vi "GUI.vi"() -> ()   [LabVIEW 2021]
uses:
  <vilib>/numeric/Random Number (Range) U64.vi
  <vilib>/numeric/sub_Random U32.vi
  <vilib>/Instr/_visa.llb/VISA Configure Serial Port (Instr).vi
panel:
  out "start sim":bool
  out "Time has Elapsed":bool
  out "Time":dbl
  out "Logging":bool caption="Time has Elapsed"
  in  "PWM":i16(slide)=1410 min=1300 max=1410 scale=1155.0..1384.0
  out "Mode":string
  in  "Mode":bool
  out "O":dbl
  out "T":dbl
  out "D":dbl
  out "I":dbl
  out "P":dbl
  out "F":dbl
  out "S":dbl
  in  "Stop Button":bool
  out "TS":dbl(slide) scale=0.0..100.0
  out "KD":dbl(slide) scale=0.0..100.0
  out "KI":dbl(slide) scale=0.0..50.0
  out "KP":dbl(slide) scale=0.0..10.0
  in  "COM Port":refnum<visa-resource-name>
  in  "Save Result":path
  out "Output PID":dbl(graph)
  out "Tacho Generator":dbl(knob) scale=0.0..1023.0
  out "SetPoint":dbl(knob) scale=0.0..1023.0
  out "Respon PID":dynamicdata(graph)
  # "ALIM SATRIA FI'I WIJAYA KUSUMA (21/483503/SV/20304)"
  # "KENDALI KECEPATAN MOTOR DC"
  # "ILHAM DWI CAHYO (21/483417/SV/20218)"
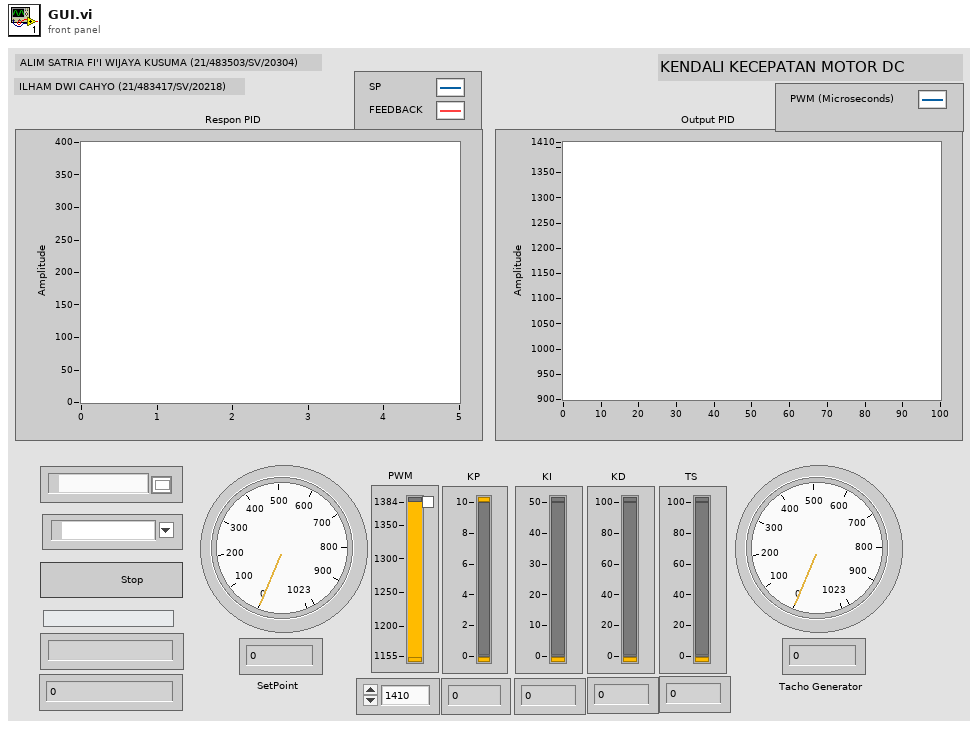
[diagram p1: front panel]
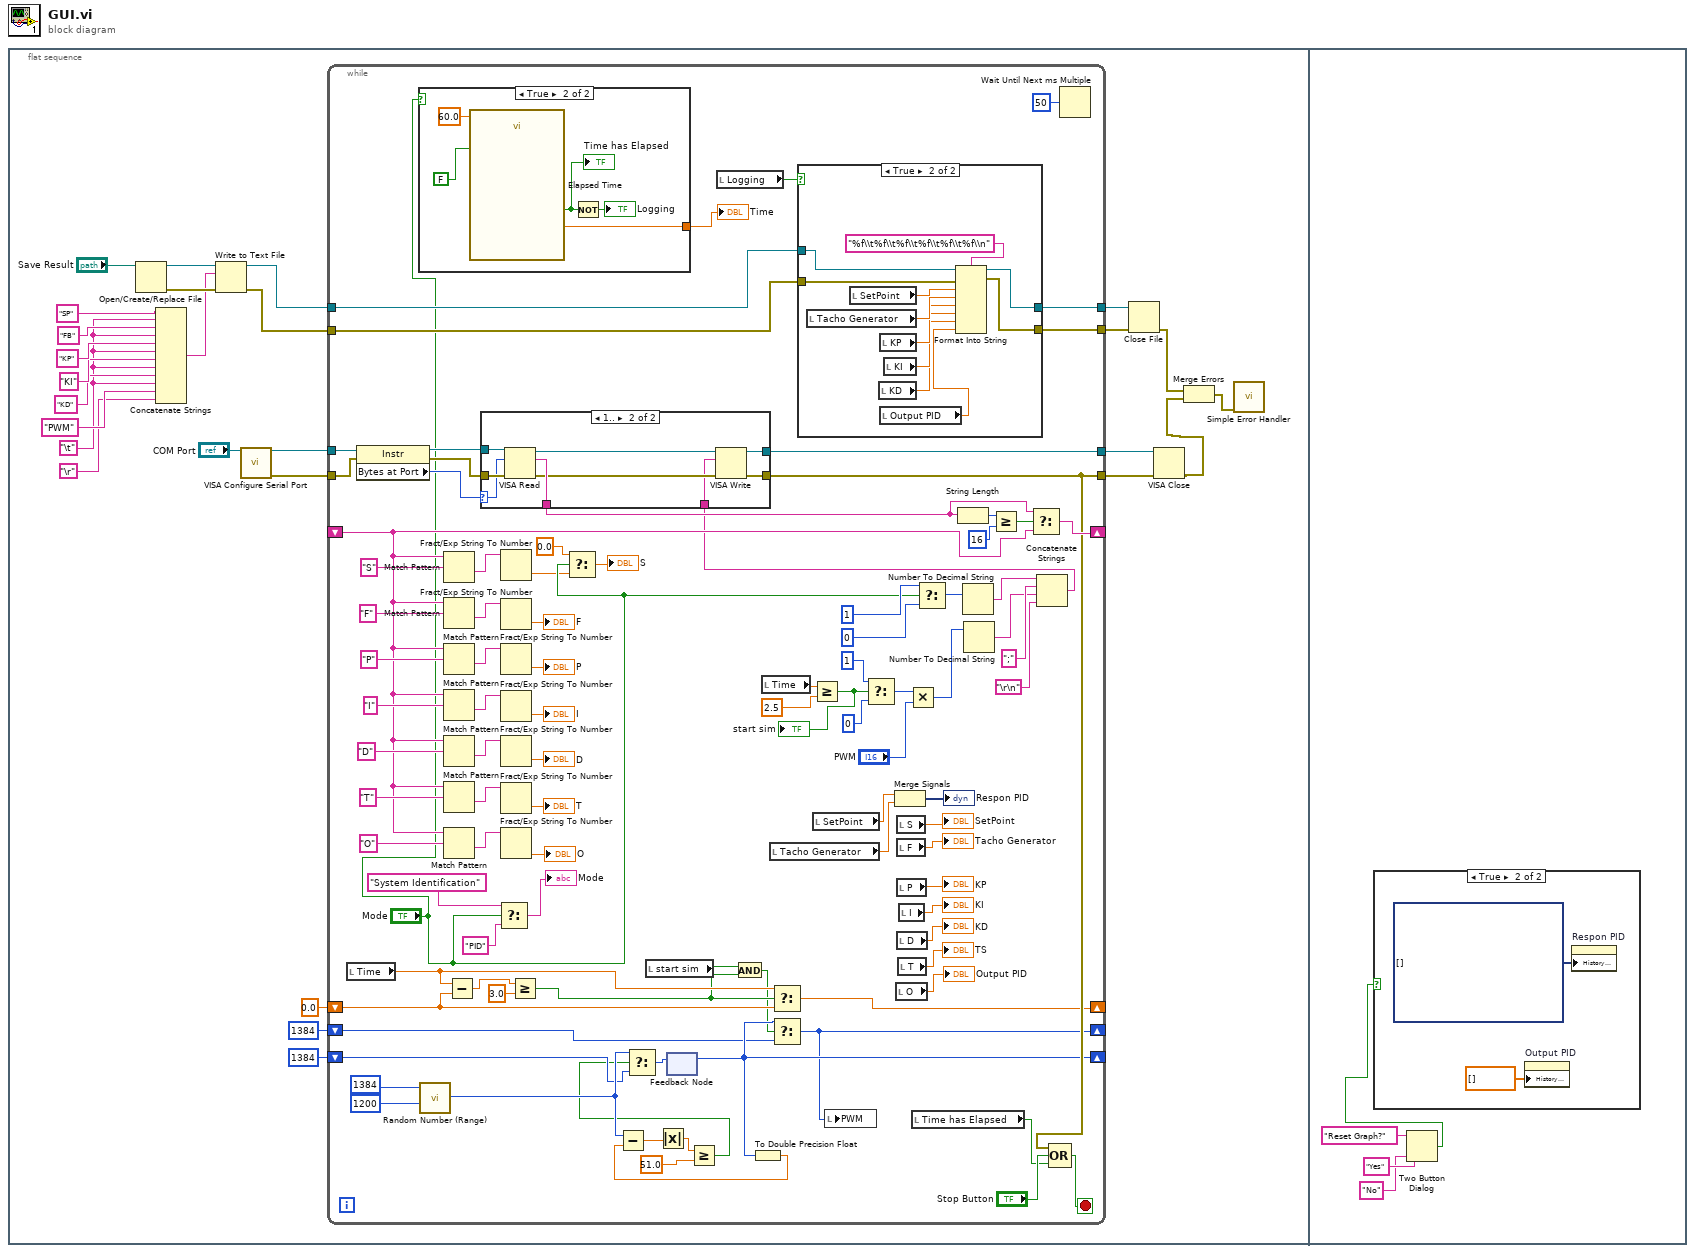
[diagram p0: block diagram]
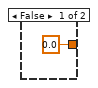
[diagram p2: hidden frame]
diagram:
  n1 = flat-sequence {
    frame #0 {
      w10 = "\t"
      n2 = Open/Create/Replace File(file path (use dialog)="Save Result") -> (refnum out=w22:refnum<file>, error out=w23:errorcluster)  [unwired: 5 in, 1 out]
      n3 = Concatenate Strings("SP", w10, "FB" ("string"), w10, "KP" ("string"), w10, "KI" ("string"), w10, "KD" ("string"), w10, "PWM", "\r") -> (w17:string)
      n4 = Write to Text File(file (use dialog)=w22, text=w17, error in=w23) -> (refnum out=w21:refnum<file>, error out=w20:errorcluster)  [unwired: 1 in, 1 out]
      n5 = call-poly "VISA Configure Serial Port"("VISA resource name"="COM Port") -> ("VISA resource name out"=w27:refnum<visa-resource-name>, "error out"=w26:errorcluster)  [unwired: 13 in]
      n6 = while {
        tunnel: w27 -> [w83]
        tunnel: w26 -> [w79]
        tunnel: [w80] -> w8
        tunnel: [w74] -> w7
        tunnel: w21 -> [w93]
        tunnel: w20 -> [w92]
        tunnel: [w91] -> w19
        tunnel: [w90] -> w18
        shift-right: [w86] -> _
        shift-left: _ -> [w85]
        shift-right: [w33] -> _
        shift-left: u64 1384 ("number") -> [w35]
        shift-right: [w40] -> _
        shift-left: 0.0 ("Time") -> [w36]
        shift-right: [w31] -> _
        shift-left: u64 1384 ("number") -> [w32]
        stop <- w124 stop-if-true
        n7 = local read "Time"() -> (w37:dbl)
        n8 = property class="Instr"(reference=w83, error in=w79) -> (reference out=w82:refnum<visa-resource-name>, error out=w81:errorcluster, "Bytes at Port"=w123:u32)
        n9 = case shown="True" "Mode" {
          tunnel: [0.0 ("Elapsed Time (s)") w127] -> w63
          frame False {
          }
          frame True {
            n10 = call "Elapsed Time"("Time Target (s)"=60.0, "Auto Reset"=FALSE) -> ("Elapsed Time (s)"=w127:dbl, "Time has Elapsed"=w130:bool)  [unwired: 10 in, 6 out]
            "Time has Elapsed" <- w130
            n11 = Not(x=w130) -> (.not. x?=→"Logging":bool)
          }
        }
        "Time" <- w63
        n12 = call-poly <vilib>:"Random Number (Range).vi"("lower bound (0)"=u64 1200, "upper bound (100)"=u64 1384) -> ("number"=w47:u64)  [unwired: 9 in]
        n13 = Match Pattern(string=w85, regular expression="S") -> (after substring=w115:string)  [unwired: 1 in, 3 out]
        n14 = Match Pattern(string=w85, regular expression="F") -> (after substring=w114:string)  [unwired: 1 in, 3 out]
        n15 = Match Pattern(string=w85, regular expression="P") -> (after substring=w113:string)  [unwired: 1 in, 3 out]
        n16 = Match Pattern(string=w85, regular expression="I") -> (after substring=w112:string)  [unwired: 1 in, 3 out]
        n17 = Match Pattern(string=w85, regular expression="D") -> (after substring=w111:string)  [unwired: 1 in, 3 out]
        n18 = Match Pattern(string=w85, regular expression="T") -> (after substring=w110:string)  [unwired: 1 in, 3 out]
        n19 = Match Pattern(string=w85, regular expression="O") -> (after substring=w109:string)  [unwired: 1 in, 3 out]
        n20 = Subtract(x=w37, y=w36) -> (x-y=w38:dbl)
        n21 = Select(t="System Identification", s="Mode", f="PID") -> (s? t:f=→"Mode":string)
        n22 = Fract/Exp String To Number(string=w115) -> (number=w52:dbl)  [unwired: 3 in, 1 out]
        n23 = Fract/Exp String To Number(string=w114) -> (number=→"F":dbl)  [unwired: 3 in, 1 out]
        n24 = Fract/Exp String To Number(string=w113) -> (number=→"P":dbl)  [unwired: 3 in, 1 out]
        n25 = Fract/Exp String To Number(string=w112) -> (number=→"I":dbl)  [unwired: 3 in, 1 out]
        n26 = Fract/Exp String To Number(string=w111) -> (number=→"D":dbl)  [unwired: 3 in, 1 out]
        n27 = Fract/Exp String To Number(string=w110) -> (number=→"T":dbl)  [unwired: 3 in, 1 out]
        n28 = Fract/Exp String To Number(string=w109) -> (number=→"O":dbl)  [unwired: 3 in, 1 out]
        n29 = Greater Or Equal?(x=w38, y=3.0) -> (x >= y?=w29:bool)
        n30 = Select(t=0.0, s="Mode", f=w52) -> (s? t:f=→"S":dbl)
        n31 = local read "start sim"() -> (w30:bool)
        n32 = feedback #1() -> (w33:u64)  [unwired: 1 in]
        n33 = local read "Logging"() -> (w64:bool)
        n34 = And(x=w30, y=w29) -> (x .and. y?=w28:bool)
        n35 = To Double Precision Float(number=w33) -> (double precision float=w43:dbl)
        n36 = Subtract(x=w47, y=w43) -> (x-y=w45:dbl)
        n37 = Absolute Value(x=w45) -> (abs(x)=w46:dbl)
        n38 = Greater Or Equal?(x=w46, y=51.0) -> (x >= y?=w34:bool)
        n39 = Select(t=w47, s=w34, f=w35) -> (s? t:f=w44:u64)
        n40 = feedback-in #1(w44) -> ()
        n41 = local read "Time"() -> (w61:dbl)
        n42 = local read "Tacho Generator"() -> (w101:dbl)
        n43 = Select(t=w37, s=w29, f=w36) -> (s? t:f=w40:dbl)
        n44 = Select(t=w33, s=w28, f=w32) -> (s? t:f=w31:u64)
        n45 = case shown="True" w64 {
          tunnel: w93 -> [w132 w143]
          tunnel: w92 -> [w131 w142]
          tunnel: [w132 w141] -> w91
          tunnel: [w131 w140] -> w90
          frame False {
          }
          frame True {
            n46 = local read "Tacho Generator"() -> (w138:dbl)
            n47 = local read "SetPoint"() -> (w139:dbl)
            n48 = local read "KD"() -> (w134:dbl)
            n49 = local read "KP"() -> (w136:dbl)
            n50 = local read "Output PID"() -> (w133:dbl)
            n51 = local read "KI"() -> (w135:dbl)
            n52 = Format Into String(format string="%f\\t%f\\t%f\\t%f\\t%f\\t%f\\n", initial string=w143, error in=w142, w139, w138, w136, w135, w134, w133) -> (resulting string=w141:refnum<file>, error out=w140:errorcluster)
          }
        }
        n53 = Greater Or Equal?(x=w61, y=2.5) -> (x >= y?=w59:bool)
        "start sim" <- w59
        n54 = local read "SetPoint"() -> (w102:dbl)
        n55 = local write "PWM"(w31) -> ()
        n56 = Select(t=i16 1, s=w59, f=i16 0) -> (s? t:f=w56:i16)
        n57 = Merge Signals(w102, w101) -> (→"Respon PID":dynamicdata)
        n58 = local read "O"() -> (→"Output PID":dbl)
        n59 = local read "S"() -> (→"SetPoint":dbl)
        n60 = local read "F"() -> (→"Tacho Generator":dbl)
        n61 = local read "P"() -> (→"KP":dbl)
        n62 = local read "D"() -> (→"KD":dbl)
        n63 = local read "T"() -> (→"TS":dbl)
        n64 = local read "I"() -> (→"KI":dbl)
        n65 = Multiply(x=w56, y="PWM") -> (x*y=w54:i16)
        n66 = local read "Time has Elapsed"() -> (w62:bool)
        n67 = Select(t=1, s="Mode", f=0) -> (s? t:f=w66:i32)
        n68 = Number To Decimal String(number=w66) -> (decimal integer string=w70:string)  [unwired: 1 in]
        n69 = Number To Decimal String(number=w54) -> (decimal integer string=w69:string)  [unwired: 1 in]
        n70 = Concatenate Strings(w70, ";", w69, "\r\n") -> (w73:string)
        n71 = case shown="1.." w123 {
          selector: w123 -> [_ w151]
          tunnel: w82 -> [w145 w154]
          tunnel: [w145 w148] -> w80
          tunnel: w81 -> [w144 w153]
          tunnel: [w144 w147] -> w74
          tunnel: [_ w152] -> w84
          tunnel: w73 -> [_ w146]
          frame 0, Default {
          }
          frame 1.. {
            n72 = VISA Read(VISA resource name=w154, byte count=w151, error in (no error)=w153) -> (VISA resource name out=w150:refnum<visa-resource-name>, read buffer=w152:string, error out=w149:errorcluster)  [unwired: 1 out]
            n73 = VISA Write(VISA resource name=w150, write buffer=w146, error in (no error)=w149) -> (VISA resource name out=w148:refnum<visa-resource-name>, error out=w147:errorcluster)  [unwired: 1 out]
          }
        }
        n74 = String Length(string=w84) -> (length=w89:i32)
        n75 = Greater Or Equal?(x=w89, y=16) -> (x >= y?=w87:bool)
        n76 = Select(t=w84, s=w87, f=w85) -> (s? t:f=w86:string)
        n77 = Compound Arithmetic op=OR(w74, "Stop Button", w62) -> (w124:bool)
        n78 = Wait Until Next ms Multiple(millisecond multiple=u32 50) -> ()  [unwired: 1 out]
      }
      n79 = Close File(refnum=w19, error in=w18) -> (error out=w6:errorcluster)  [unwired: 1 out]
      n80 = VISA Close(VISA resource name=w8, error in (no error)=w7) -> (error out=w5:errorcluster)
      n81 = Merge Errors(w6, w5) -> (w4:errorcluster)
      n82 = call <vilib>:"Simple Error Handler.vi"("error in (no error)"=w4) -> ()  [unwired: 4 in, 5 out]
    }
    frame #1 {
      n83 = Two Button Dialog(message="Reset Graph?", 1:"No" ("F button name (\"Cancel\")"), 2:"Yes" ("T button name (\"OK\")")) -> (T button?=w155:bool)
      n84 = case shown="True" w155 {
        frame False {
        }
        frame True {
          n85 = property on="Output PID" class="WFChart (strict)"("History Data"=dbl[] []) -> ()  [unwired: 2 in, 2 out]
          n86 = property on="Respon PID" class="WFChart (strict)"("History Data"=dynamicdata[] []) -> ()  [unwired: 2 in, 2 out]
        }
      }
    }
  }
